vi "获取图像.vi"(0 "DevCfgGet":cluster{"pid":u32, "vid":u32, "ser_num":u64}[](array[cluster]), 1 "设备列表":i32[](array[numeric]), 2 "设备":u16(ring) items=["设备1_22592_3034"], 3 "camera_stream_info":T1(array[cluster]), 4 "分辨率":string(combo), 5 "FPS":u32, 7 "error in":errorcluster) -> (20 "内部出图返回值":i32, 27 "error out":errorcluster)   [LabVIEW 2016]
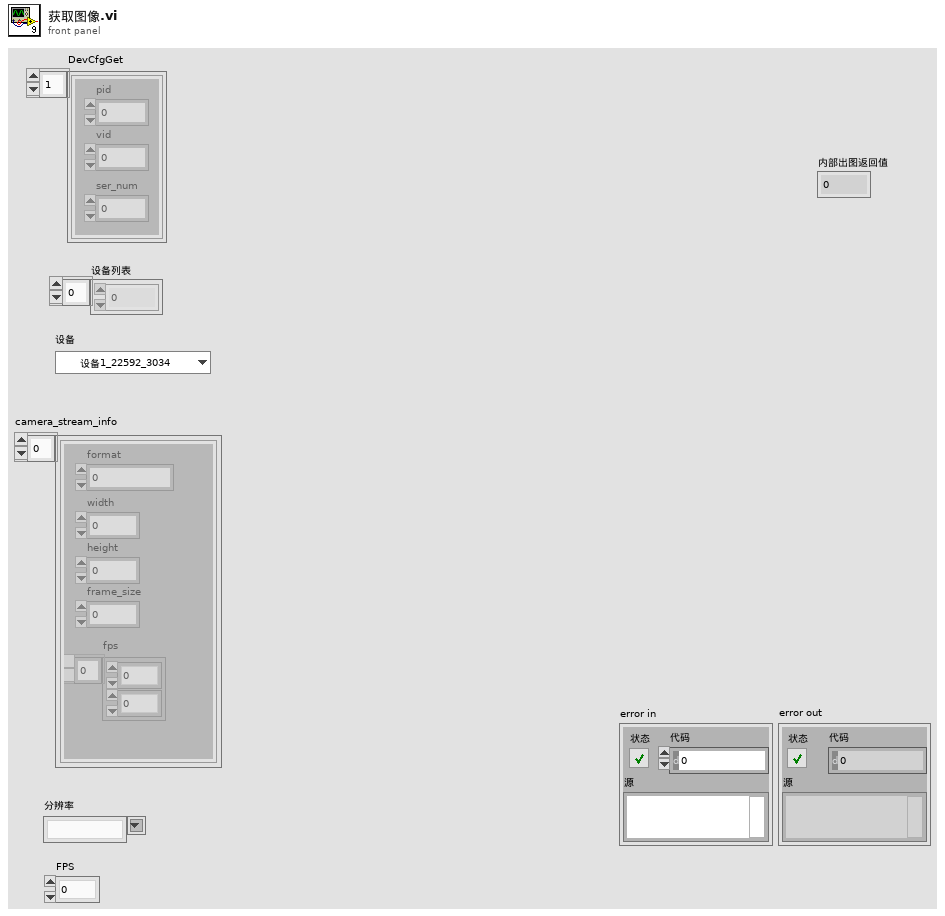
[diagram p1: front panel]
types:
  T1 = cluster{"format":u64, "width":u32, "height":u32, "frame_size":u32, "fps":u32[]}[]
  T2 = cluster{"DevCfg":cluster{"pid":u32, "vid":u32, "ser_num":u64}, "format":u64, "width":u32, "height":u32, "frame_size":u32, "fps":u32, "timeout 2":u32}
  T3 = cluster{"format":u64, "width":u32, "height":u32, "frame_size":u32, "fps":u32[]}
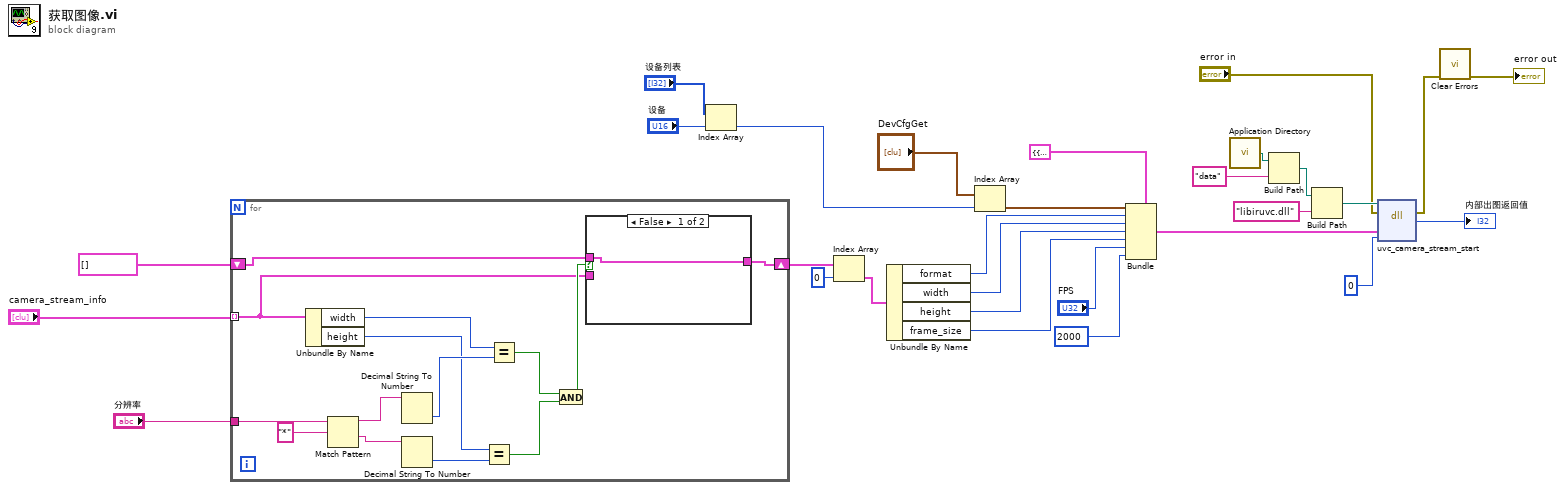
[diagram p0: block diagram]
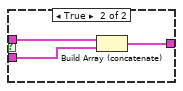
[diagram p2: hidden frame]
diagram:
  n1 = for {
    tunnel: "camera_stream_info" -> [w30] mode=indexing
    tunnel: "分辨率" -> [w43]
    shift-right: [w32] -> w7
    shift-left: T1 [] ("camera_stream_info[] 2") -> [w33]
    n2 = Unbundle By Name(w30) -> ("width"=w39:u32, "height"=w37:u32)
    n3 = Match Pattern(string=w43, regular expression="*") -> (before substring=w41:string, after substring=w40:string)  [unwired: 1 in, 2 out]
    n4 = Decimal String To Number(string=w41) -> (number=w38:i32)  [unwired: 2 in, 1 out]
    n5 = Decimal String To Number(string=w40) -> (number=w36:i32)  [unwired: 2 in, 1 out]
    n6 = Equal?(x=w37, y=w36) -> (x = y?=w35:bool)
    n7 = Equal?(x=w39, y=w38) -> (x = y?=w34:bool)
    n8 = And(x=w34, y=w35) -> (x .and. y?=w31:bool)
    n9 = case shown="False" w31 {
      tunnel: w33 -> [w44 w47]
      tunnel: [w44 w46] -> w32
      tunnel: w30 -> [_ w45]
      frame False {
      }
      frame True {
        n10 = Build Array (concatenate)(w47, w45) -> (w46:T1)
      }
    }
  }
  n11 = Index Array(array="设备列表", index="设备") -> (element=w21:i32)
  n12 = Index Array(array=w7, index=0) -> (element=w5:T3)
  n13 = Unbundle By Name(w5) -> ("format"=w4:u64, "width"=w3:u32, "height"=w2:u32, "frame_size"=w1:u32)
  n14 = Index Array(array="DevCfgGet", index=w21) -> (element=w29:cluster{"pid":u32, "vid":u32, "ser_num":u64})
  n15 = Bundle(cluster=T2 {"DevCfg"={"pid"=0, "vid"=0, "ser_num"=0}, "format"=0, "width"=0, "height"=0, "frame_size"=0, "fps"=0, "timeout 2"=0} ("CameraParam"), "DevCfg"=w29, "format"=w4, "width"=w3, "height"=w2, "frame_size"=w1, "fps"="FPS", "timeout 2"=2000) -> (w28:T2)
  n16 = call <vilib>:"Application Directory.vi"() -> ("Application Directory"=w23:path)
  n17 = Build Path(base path=w23, name or relative path="data") -> (appended path=w25:path)
  n18 = Build Path(base path=w25, name or relative path="libiruvc.dll") -> (appended path=w22:path)
  n19 = dll-call lib="D:/libiruvc_0.3.3/windows/x64/dll/libiruvc.dll" fn="uvc_camera_stream_start"(path in=w22, error in="error in", "CameraParam"=w28, "usr_func"=u8 0) -> (error out=w14:errorcluster, "return type"=→"内部出图返回值":i32)  [unwired: 3 in, 1 out]
  n20 = call <vilib>:"Clear Errors.vi"("error in (no error)"=w14) -> ("error out"=→"error out":errorcluster)  [unwired: 5 in, 1 out]
